vi "Run.vi"(8 "error in (no error)":errorcluster, 9 "s on last turn":dbl, 10 "Maze (0: Empty, -1: Enemy. >0: Teammate":i32[][](array[numeric]), 11 "Scout In":refnum<class "Protector.lvclass">) -> (0 "error out":errorcluster, 1 "Direction":T1, 2 "Action":T2, 3 "Scout Out":refnum<class "Protector.lvclass">, 4 "Replicated":refnum<class "Runner.lvclass">)   [LabVIEW 2014, in "Protector.lvclass"]
uses:
  Protector.lvclass
  Action Enum.ctl
  Direction Enum.ctl
  Runner.lvclass
  Mother/Attack Options.ctl
  Mother/Mother.lvclass/Mother.ctl
  Mother/Mother.lvclass
  SquareBattle.lvclass
panel:
  out "Map":i32[](array[numeric])
  in  "Status":string
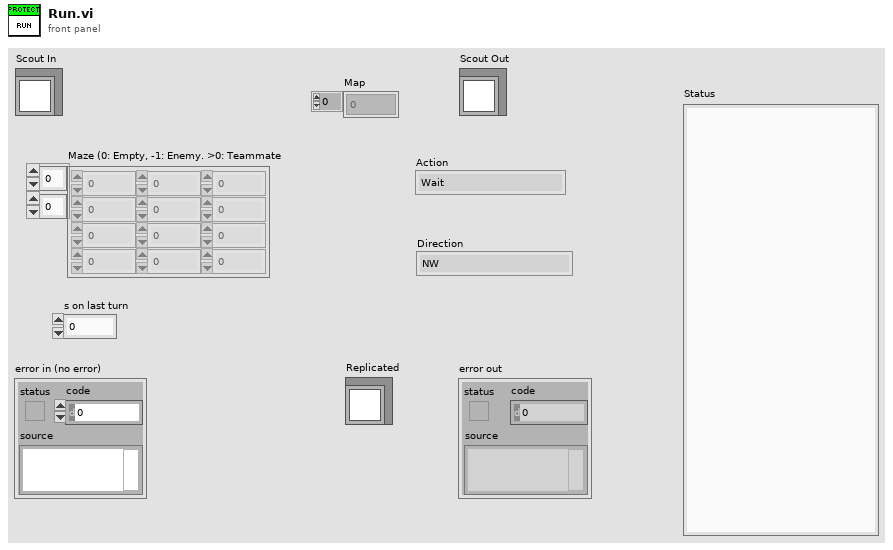
[diagram p1: front panel]
types:
  T1 = typedef "SquareBattle.lvclass/Direction Enum.ctl" = enum16{"NW", "N", "NE", "E", "SE", "S", "SW", "W"}
  T2 = typedef "SquareBattle.lvclass/Action Enum.ctl" = enum16{"Wait", "Move", "Attack", "Replicate"}
  T3 = typedef "Attack Options.ctl" = enum16{"Attack", "Run", "Distract"}
  T4 = typedef "Kamikaze DVR.ctl" = refnum<data-value>
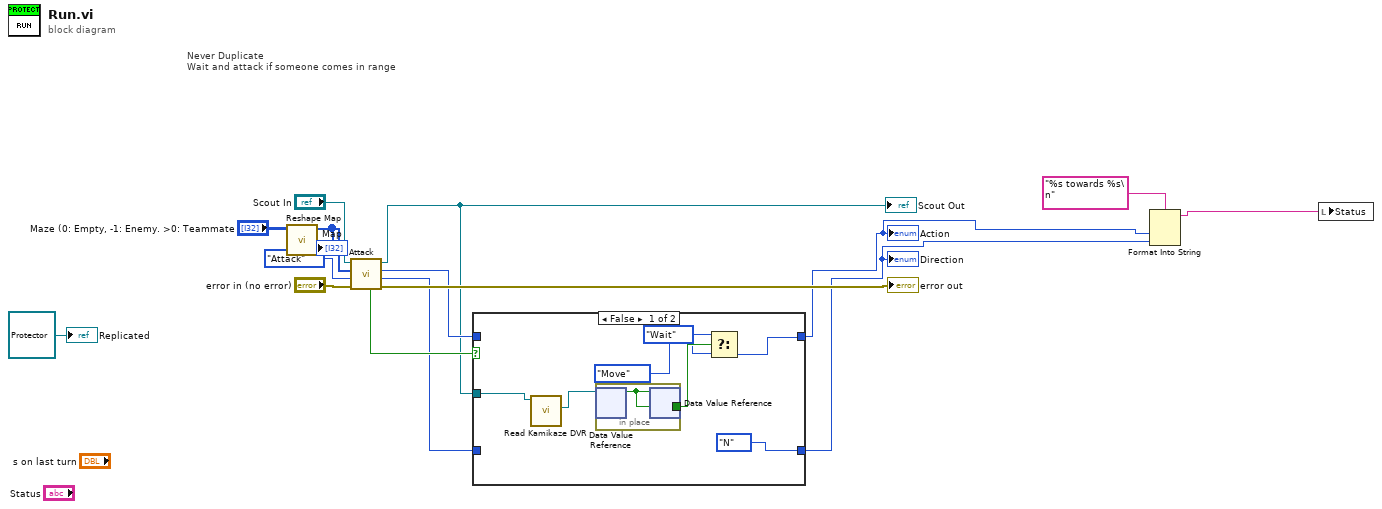
[diagram p0: block diagram]
diagram:
  # "Never Duplicate\nWait and attack if someone comes in range"
  n1 = call "Reshape Map.vi"("Maze (0: Empty, -1: Enemy. >0: Teammate"="Maze (0: Empty, -1: Enemy. >0: Teammate") -> ("Map"=w10:i32[])  [unwired: 9 in, 1 out]
  "Map" <- w10
  n2 = call "Attack.vi"("error in (no error)"="error in (no error)", "Attack?"=Attack_Options."Attack", "Maze (0: Empty, -1: Enemy. >0: Teammate"=w10, "Mother in"="Scout In") -> ("error out"=→"error out":errorcluster, "Direction"=w3:T1, "Action"=w5:T2, "Mother out"=w1:refnum<class "Protector.lvclass">, "Enemy Found?"=w6:bool)  [unwired: 2 in, 1 out]
  "Scout Out" <- w1
  n3 = case shown="False" w6 {
    tunnel: w5 -> [_ w25]
    tunnel: w3 -> [_ w24]
    tunnel: [w18 w25] -> w4
    tunnel: [Direction_Enum."N" ("Direction") w24] -> w2
    tunnel: w1 -> [w22 _]
    frame False {
      n4 = call "Read Kamikaze DVR.vi"("Mother in"=w22) -> ("Kamikaze DVR"=w21:T4)  [unwired: 8 in, 2 out]
      n5 = in-place {
        in-place-border: [w23] -> w17
        n6 = in-place-dvr #1(w21) -> (w23:bool)  [unwired: 1 out]
        n7 = in-place-dvr #1(w23) -> ()  [unwired: 2 out]
      }
      n8 = Select(t=Action_Enum."Move" ("Action"), s=w17, f=Action_Enum."Wait" ("t")) -> (s? t:f=w18:T2)
    }
    frame True {
    }
  }
  "Action" <- w4
  "Direction" <- w2
  n9 = Format Into String(format string="%s towards %s\n", w4, w2) -> (resulting string=w7:string)  [unwired: 2 in, 1 out]
  n10 = local write "Status"(w7) -> ()
  "Replicated" <- refnum<class "Protector.lvclass"> refnum ("Replicated")
